vi "Get all VIs in Project.vi"(8 "error in (no error)":errorcluster, 10 "Path":path, 11 "Coverage Analyzer in":refnum<class "Coverage Analyzer.lvclass">) -> (0 "error out":errorcluster, 2 "VIs":set{path}(c389), 3 "Coverage Analyzer out":refnum<class "Coverage Analyzer.lvclass">)   [LabVIEW 2020, in "Coverage Analyzer.lvclass"]
uses:
  Coverage Analyzer.lvclass
  2fa7b275-f75d-4bcf-8530-71b3ed265666.vi
  Coverage Analyzer.lvclass/Coverage Analyzer.ctl
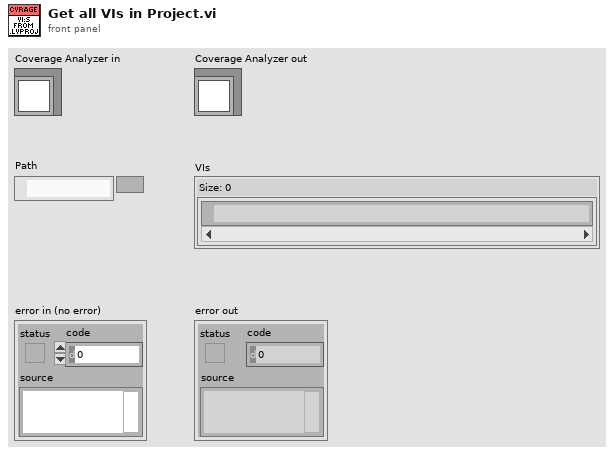
[diagram p1: front panel]
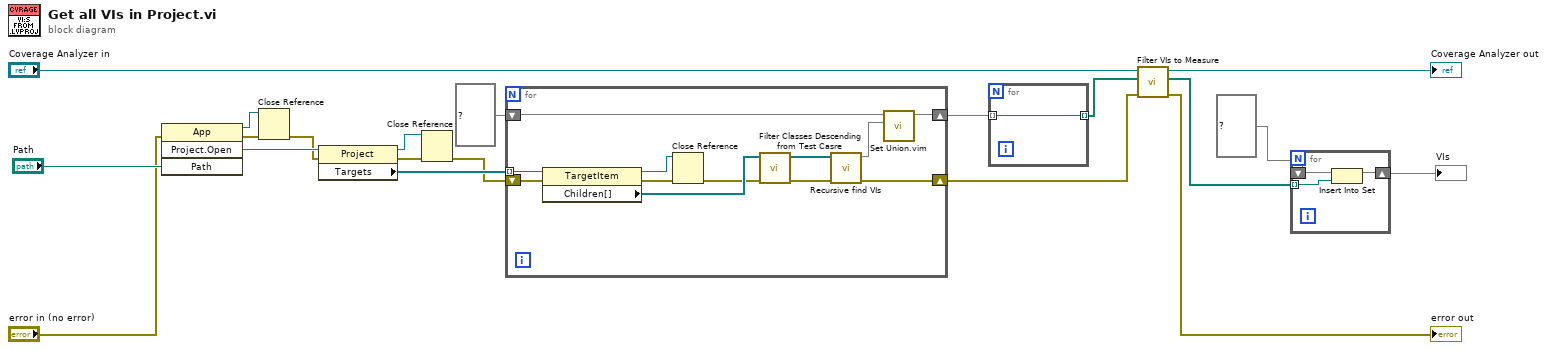
[diagram p0: block diagram]
diagram:
  n1 = invoke class="App" method="Project.Open"(error in="error in (no error)", "Path"="Path") -> (reference out=w11:refnum<vi>, error out=w16:errorcluster, "Project:Open"=w19:refnum<vi>)  [unwired: 2 in, 1 out]
  n2 = Close Reference(reference=w11, error in (no error)=w16) -> (error out=w12:errorcluster)
  n3 = property class="Project"(reference=w19, error in=w12) -> (reference out=w13:refnum<vi>, error out=w17:errorcluster, "Targets"=w18:refnum<vi>[])
  n4 = Close Reference(reference=w13, error in (no error)=w17) -> (error out=w14:errorcluster)
  n5 = for {
    tunnel: w18 -> [w32] mode=indexing
    shift-right: [w29] -> w7
    shift-left: w14 -> [w30]
    shift-right: [w25] -> w5
    shift-left: set{path} {} ("VIs") -> [w27]
    n6 = property class="TargetItem"(reference=w32, error in=w30) -> (reference out=w28:refnum<vi>, error out=w31:errorcluster, "Children[]"=w24:refnum<vi>[])
    n7 = Close Reference(reference=w28, error in (no error)=w31) -> (error out=w22:errorcluster)
    n8 = call "Filter Classes Descending from Test Casre.vi"("error in (no error)"=w22, "Project Items"=w24) -> ("error out"=w21:errorcluster, "Project Items out"=w23:refnum<vi>[])  [unwired: 8 in]
    n9 = call "Recursive find VIs.vi"("error in (no error)"=w21, "Project Items"=w23) -> ("error out"=w29:errorcluster, "VIs"=w26:set{path})  [unwired: 8 in]
    n10 = call "Set Union.vim"("set 2"=w26, "set 1"=w27) -> ("union"=w25:set{path})  [unwired: 9 in]
  }
  n11 = for {
    tunnel: w5 -> [w33] mode=indexing
    tunnel: [w33] -> w4 mode=indexing
  }
  n12 = call "Filter VIs to Measure.vi"("error in (no error)"=w7, "VI Paths"=w4, "Coverage Analyzer in"="Coverage Analyzer in") -> ("error out"=→"error out":errorcluster, "Filtered VI Paths"=w1:path[], "Coverage Analyzer out"=→"Coverage Analyzer out":refnum<class "Coverage Analyzer.lvclass">)  [unwired: 6 in]
  n13 = for {
    shift-right: [w35] -> w2
    shift-left: set{path} {} ("VIs") -> [w36]
    tunnel: w1 -> [w34] mode=indexing
    n14 = Insert Into Set(10:w34, 11:w36) -> (3:w35:set{path})  [unwired: 1 out]
  }
  "VIs" <- w2
